vi "Set Node IDs.vi"(8 "error in":errorcluster, 10 "FolderIDs":T2, 11 "Panel in":refnum<class "Panel.lvclass">) -> (0 "error out":errorcluster, 3 "Panel out":refnum<class "Panel.lvclass">)   [LabVIEW 2021, in "Panel.lvlib" / "Panel.lvclass"]
uses:
  Panel.lvclass
  <vilib>/OPCUA/controls/OPC UA Server Refnum.ctl
  Panel.lvclass/Panel.ctl
  <vilib>/OPCUA/controls/Data Type.ctl
  Station/Station Actor/Station.lvclass
  <vilib>/OPCUA/NI OPC UA Server.lvlib
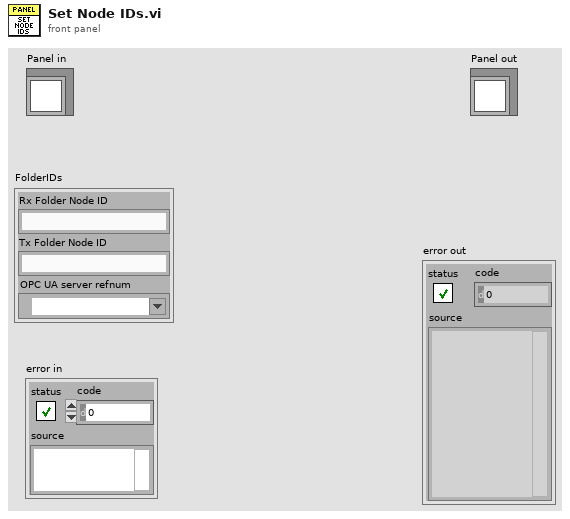
[diagram p1: front panel]
types:
  T1 = typedef "OPC UA Server Refnum.ctl" = refnum<k21>
  T2 = cluster{"Rx Folder Node ID":string, "Tx Folder Node ID":string, "OPC UA server refnum":T1}
  T3 = typedef "Data Type.ctl" = u16
  T4 = cluster{"name":string, "data type":T3, "access level":u16, "description":string}
  T5 = typedef "NodeId.ctl" = string
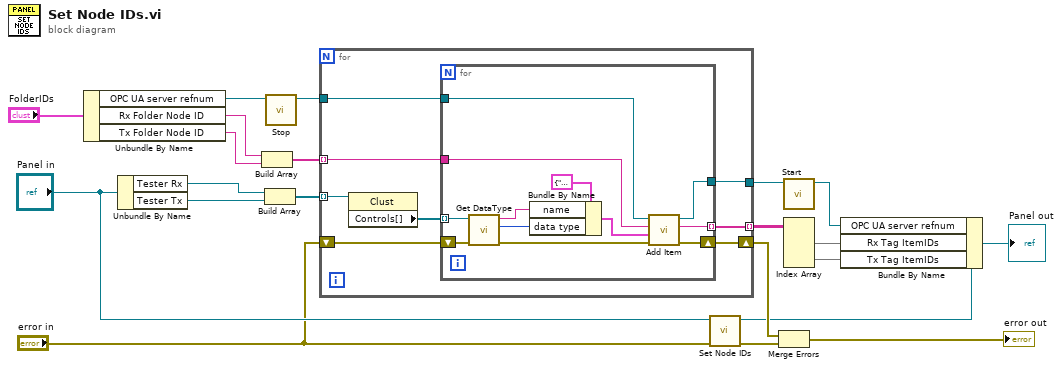
[diagram p0: block diagram]
diagram:
  n1 = Unbundle By Name("FolderIDs") -> ("OPC UA server refnum"=w6:T1, "Rx Folder Node ID"=w12:string, "Tx Folder Node ID"=w11:string)
  n2 = Unbundle By Name("Panel in") -> ("Tester Rx"=w14:refnum<vi>, "Tester Tx"=w13:refnum<vi>)
  n3 = Build Array(w12, w11) -> (w19:string[])
  n4 = Build Array(w14, w13) -> (w15:refnum<vi>[])
  n5 = call <vilib>:"Stop.vi"("OPC UA server refnum in"=w6) -> ("OPC UA server refnum out"=w5:T1)  [unwired: 9 in, 1 out]
  n6 = for {
    tunnel: w15 -> [w27] mode=indexing
    tunnel: w19 -> [w26] mode=indexing
    tunnel: [w25] -> w16 mode=indexing
    shift-right: [w28] -> w7
    shift-left: "error in" -> [w29]
    tunnel: w5 -> [w23]
    tunnel: [w22] -> w4
    n7 = property class="Clust"(reference=w27) -> ("Controls[]"=w24:refnum<vi>[])  [unwired: 1 in, 2 out]
    n8 = for {
      tunnel: w26 -> [w41]
      shift-right: [w40] -> w28
      shift-left: w29 -> [w35]
      tunnel: [w39] -> w25 mode=indexing
      tunnel: w24 -> [w36] mode=indexing
      tunnel: w23 -> [w31]
      tunnel: [w30] -> w22
      n9 = call "Get DataType.vi"("error in (no error)"=w35, "reference"=w36) -> ("error out"=w33:errorcluster, "data type"=w32:T3, "Name"=w34:string)  [unwired: 7 in]
      n10 = Bundle By Name(cluster=T4 {"name"="", "data type"=1, "access level"=3, "description"=""} ("item"), "name"=w34, "data type"=w32) -> (w37:T4)
      n11 = call <vilib>:"Add Item.vi"("error in (no error)"=w33, "item"=w37, "parent folder node ID"=w41, "OPC UA server refnum in"=w31) -> ("error out"=w40:errorcluster, "item node ID"=w39:T5, "OPC UA server refnum out"=w30:T1)  [unwired: 3 in, 1 out]
    }
  }
  n12 = call-parent "Set Node IDs.vi"("error in (no error)"="error in", "Station in"="Panel in") -> ("error out"=w21:errorcluster, "Station out"=w2:refnum<class "Panel.lvclass">)  [unwired: 8 in]
  n13 = Merge Errors(w7, w21) -> (→"error out":errorcluster)
  n14 = call <vilib>:"Start.vi"("OPC UA server refnum in"=w4) -> ("OPC UA server refnum out"=w3:T1)  [unwired: 8 in, 2 out]
  n15 = Index Array(array=w16) -> (element #1=w17:T5[], element #2=w18:T5[])  [unwired: 4 in]
  n16 = Bundle By Name(cluster=w2, "OPC UA server refnum"=w3, "Rx Tag ItemIDs"=w17, "Tx Tag ItemIDs"=w18) -> (→"Panel out":refnum<class "Panel.lvclass">)
